vi "CallPopupDialog.vi"(10 "Open/Close":bool, 11 "Enum":enum16{"Finished", "Pass", "Fail", "Error"}(ring)) -> ()   [LabVIEW 2018]
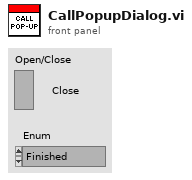
[diagram p1: front panel]
types:
  T1 = enum32{"Bad", "Idle", "Run top level", "Running"}
  T2 = enum32{"Invalid", "Standard", "Closed", "Hidden", "Minimized", "Maximized"}
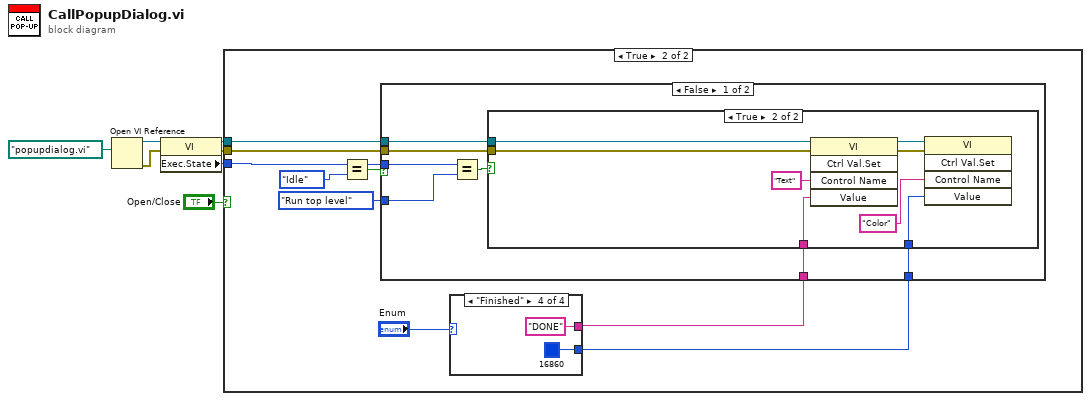
[diagram p0: block diagram]
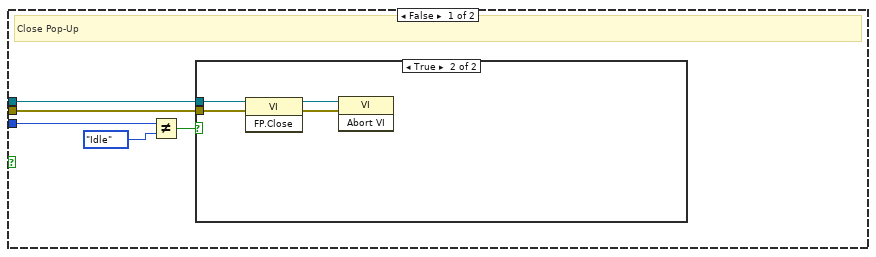
[diagram p2: hidden frame]
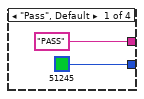
[diagram p4: hidden frame]
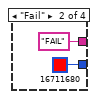
[diagram p5: hidden frame]
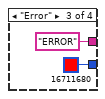
[diagram p6: hidden frame]
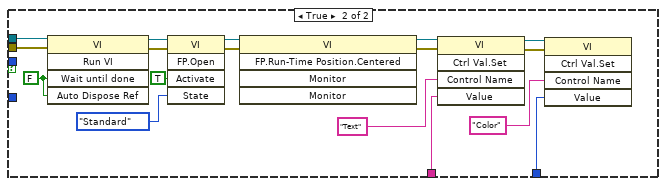
[diagram p8: hidden frame]
diagram:
  n1 = Open VI Reference(vi path=path "popupdialog.vi") -> (vi reference=w6:refnum<vi>, error out=w5:errorcluster)  [unwired: 5 in]
  n2 = property class="VI"(reference=w6, error in=w5) -> (reference out=w3:refnum<vi>, error out=w2:errorcluster, "Exec.State"=w4:T1)
  n3 = case shown="True" "Open/Close" {
    tunnel: w4 -> [w12 w18]
    tunnel: w3 -> [w10 w24]
    tunnel: w2 -> [w9 w23]
    frame False {
      # "Close Pop-Up"
      n4 = Not Equal?(x=w12, y=T1."Idle" ("Exec.State")) -> (x != y?=w8:bool)
      n5 = case shown="True" w8 {
        tunnel: w10 -> [_ w16]
        tunnel: w9 -> [_ w15]
        frame False {
        }
        frame True {
          n6 = invoke class="VI" method="FP.Close"(reference=w16, error in=w15) -> (reference out=w14:refnum<vi>, error out=w13:errorcluster)  [unwired: 1 in, 1 out]
          n7 = invoke class="VI" method="Abort VI"(reference=w14, error in=w13) -> ()  [unwired: 1 in, 3 out]
        }
      }
    }
    frame True {
      n8 = Equal?(x=w18, y=T1."Idle" ("Execution:State")) -> (x = y?=w22:bool)
      n9 = case shown="\"Finished\"" "Enum" {
        tunnel: ["PASS" "FAIL" "ERROR" "DONE"] -> w20
        tunnel: [u32 51245 u32 16711680 u32 16711680 u32 16860] -> w19
        frame "Pass", Default {
        }
        frame "Fail" {
        }
        frame "Error" {
        }
        frame "Finished" {
        }
      }
      n10 = case shown="False" w22 {
        tunnel: w24 -> [w38 w65]
        tunnel: w23 -> [w37 w64]
        tunnel: w20 -> [w35 w50]
        tunnel: w19 -> [w36 w49]
        tunnel: w18 -> [w40 _]
        tunnel: T1."Run top level" ("Execution:State") -> [w39 _]
        frame False {
          n11 = Equal?(x=w40, y=w39) -> (x = y?=w34:bool)
          n12 = case shown="True" w34 {
            tunnel: w38 -> [_ w48]
            tunnel: w37 -> [_ w47]
            tunnel: w36 -> [_ w42]
            tunnel: w35 -> [_ w41]
            frame False {
            }
            frame True {
              n13 = invoke class="VI" method="Ctrl Val.Set"(reference=w48, error in=w47, "Control Name"="Text", "Value"=w41) -> (reference out=w46:refnum<vi>, error out=w45:errorcluster)  [unwired: 1 in, 3 out]
              n14 = invoke class="VI" method="Ctrl Val.Set"(reference=w46, error in=w45, "Control Name"="Color", "Value"=w42) -> ()  [unwired: 1 in, 5 out]
            }
          }
        }
        frame True {
          w63 = FALSE ("Wait Until Done")
          n15 = invoke class="VI" method="Run VI"(reference=w65, error in=w64, "Wait until done"=w63, "Auto Dispose Ref"=w63) -> (reference out=w62:refnum<vi>, error out=w61:errorcluster)  [unwired: 1 in, 3 out]
          n16 = invoke class="VI" method="FP.Open"(reference=w62, error in=w61, "Activate"=TRUE ("Activate?"), "State"=T2."Standard") -> (reference out=w58:refnum<vi>, error out=w57:errorcluster)  [unwired: 1 in, 3 out]
          n17 = invoke class="VI" method="FP.Run-Time Position.Centered"(reference=w58, error in=w57) -> (reference out=w56:refnum<vi>, error out=w55:errorcluster)  [unwired: 3 in, 3 out]
          n18 = invoke class="VI" method="Ctrl Val.Set"(reference=w56, error in=w55, "Control Name"="Text", "Value"=w50) -> (reference out=w53:refnum<vi>, error out=w51:errorcluster)  [unwired: 1 in, 3 out]
          n19 = invoke class="VI" method="Ctrl Val.Set"(reference=w53, error in=w51, "Control Name"="Color", "Value"=w49) -> ()  [unwired: 1 in, 5 out]
        }
      }
    }
  }
